vi "LV String to PLC String.vi"(10 "StringLength In PLC":i32=50, 11 "Normal String IN LV":string) -> (3 "Full String In PLC":string)   [LabVIEW 2021]
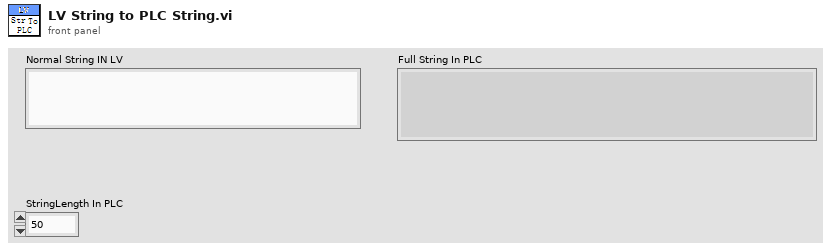
[diagram p1: front panel]
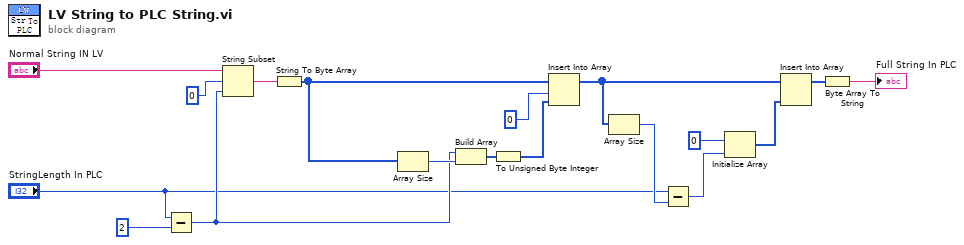
[diagram p0: block diagram]
diagram:
  n1 = Subtract(x="StringLength In PLC", y=2) -> (x-y=w7:i32)
  n2 = String Subset(string="Normal String IN LV", offset (0)=0, length (rest)=w7) -> (substring=w9:string)
  n3 = String To Byte Array(string=w9) -> (unsigned byte array=w1:u8[])
  n4 = Array Size(array=w1) -> (size(s)=w8:i32)
  n5 = Build Array(w7, w8) -> (w6:i32[])
  n6 = To Unsigned Byte Integer(number=w6) -> (unsigned 8bit integer=w5:u8[])
  n7 = Insert Into Array(array=w1, index=0, new element=w5) -> (w17:u8[])
  n8 = Array Size(array=w17) -> (size(s)=w14:i32)
  n9 = Subtract(x="StringLength In PLC", y=w14) -> (x-y=w15:i32)
  n10 = Initialize Array(u8 0 ("element"), w15) -> (w18:u8[])
  n11 = Insert Into Array(array=w17, new element=w18) -> (w12:u8[])  [unwired: 1 in]
  n12 = Byte Array To String(unsigned byte array=w12) -> (string=→"Full String In PLC":string)
